vi "niDTS BT UTIL TV to Parameters.vi"(10 "BT Tx Parameters":T2={"Channel"=0, "Data Rate "=1, "Dut Tx Power"=0.0, "External Attenuation (dB)"=[0.0, 0.0, 0.0, 0.0], "Auto Level"=FALSE, "Packet type"=enum."DH1", "Payload Pattern"=enum."PN9", "Burst Sync"=enum."PREamble", "BD ADDRESS"=0, "Packet Length, bytes"=37, "ModAcc Measurement Paramaters"={"ModAcc Enable"=FALSE, "CFO Enable"=FALSE, "Character Select"=enum."DF1", "Averages"=1, "Averaging Mode"=enum."RMS", "Measurement Length"=-1, "Measurement Offset"=0}, "OBW Measurement Parameters"={"OBW Enable"=FALSE, "OBW Averages"=1, "Averaging Type"=enum."RMS", "Measurement Interval Mode"=enum."AUTO", "Measurement Interval Length (sec)"=0.005}, "TXP Measurement Parameters"={"TXP Power Enable"=FALSE, "TXP Averages"=1, "Averaging Type"=enum."RMS"}, "IBE  Measurement Parameters"={"IBE Enable"=FALSE, "IBE Averages"=1, "Averaging Type"=enum."RMS", "Numbe of Channels"=11, "Channel Mode"=enum."Centered", "Measurement Interval Mode"=enum."AUTO", "Measurement Interval Length (sec)"=0.005}, "Trace Enable"=FALSE, "Trigger"={"MinQuietTimeDuration (sec)"=0.0001, "TriggerDelay (sec)"=0.0, "TriggerEdge"=enum."RISing", "TriggerSource"=enum."RF0", "TriggerThreshold (dB)"=-20.0, "TriggerTimeout (sec)"=10.0}} {"BD ADDRESS" max=16777215 format="%.0x"}) -> (2 "niDTS BT DUT Parameters":T1={"Channel"=0, "Pattern"=enum."PN9", "Packet type"=enum."DH1", "Power"=0.0, "Report Period (ms)"=0.0, "BD Address"=0, "Data Rate"=enum."1", "Number of Packets"=1500, "Packet Length, bytes"=37} {"BD Address" format="%x"})   [LabVIEW 2015, in "niDTS BT.lvlib"]
uses:
  niDTS BT.lvlib
  Tests/Tx Test/Includes/niDTS BT Tx Test INC Parameters.ctl
  Includes/niDTS BT INC Packet Type.ctl
  Tests/Tx Test/Includes/niDTS BT Tx Test INC BD Payload Data.ctl
  Tests/Tx Test/Includes/niDTS BT Tx Test INC Modulation Characteristics.ctl
  Includes/niDTS BT INC OBW Measurement Parameters.ctl
  Includes/niDTS BT INC TXP Measurement Parameters.ctl
  Tests/EDR Tx Test/Includes/niDTS BT INC EDR IBE Measurement Parameters.ctl
  Includes/niDTS BT DUT INC Trigger.ctl
  Includes/niDTS BT DUT INC Parameters.ctl
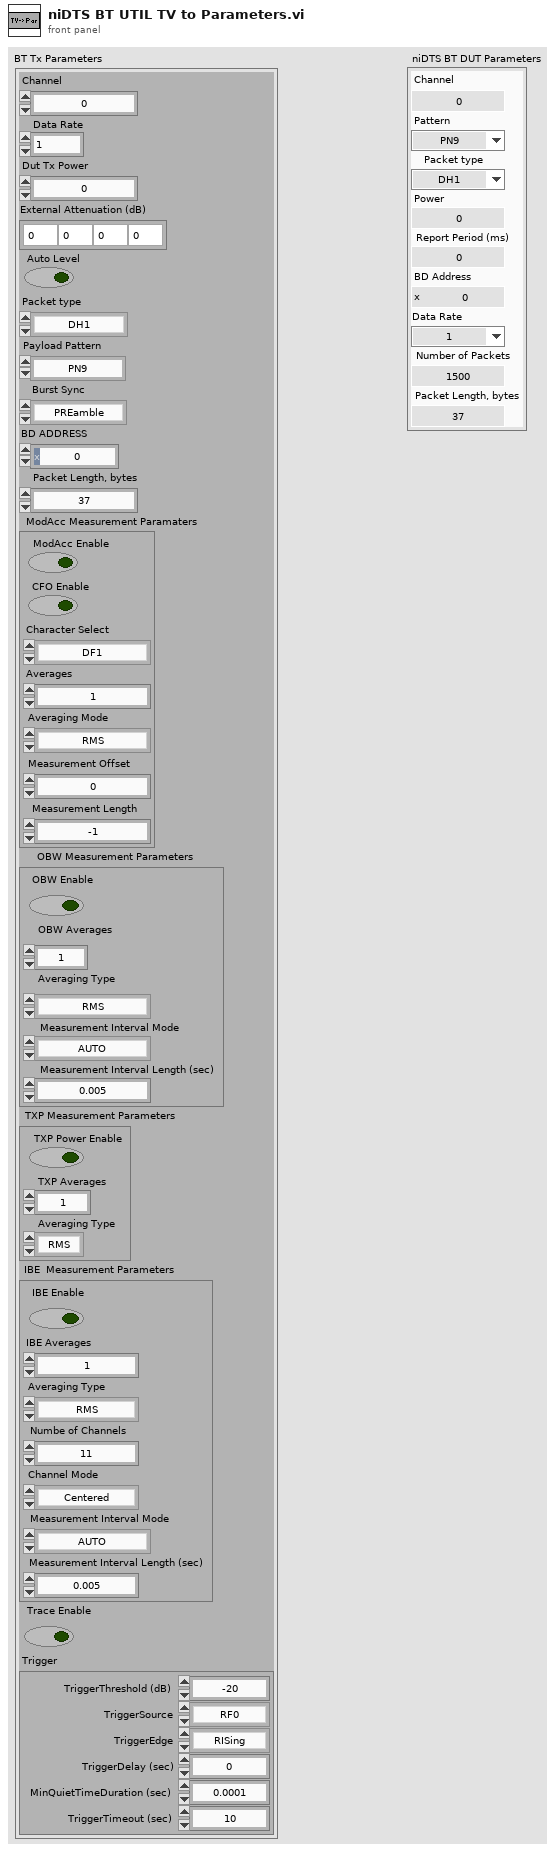
[diagram p1: front panel]
types:
  T1 = typedef "niDTS BT.lvlib/niDTS BT DUT INC Parameters.ctl" = cluster{"Channel":i32, "Pattern":enum16{"0", "1", "01", "00001111", "PN9"}, "Packet type":enum16{"NULL", "POLL", "FHS", "DM1", "DH1", "HV1", "HV2", "HV3", "EV3", "DV", "AUX1", "DM3", "DH3", "EV4", "EV5", "DM5", "DH5", "LE-TP"}, "Power":dbl, "Report Period (ms)":dbl, "BD Address":i64, "Data Rate":enum16{"1", "2", "3"}, "Number of Packets":i32, "Packet Length, bytes":i32}
  T2 = typedef "niDTS BT.lvlib/niDTS BT Tx Test INC Parameters.ctl" = cluster{"Channel":i32, "Data Rate ":i32, "Dut Tx Power":dbl, "External Attenuation (dB)":dbl[], "Auto Level":bool, "Packet type":T3, "Payload Pattern":T4, "Burst Sync":enum16{"NONE", "PREamble"}, "BD ADDRESS":u32, "Packet Length, bytes":i32, "ModAcc Measurement Paramaters":cluster{"ModAcc Enable":bool, "CFO Enable":bool, "Character Select":T5, "Averages":i32, "Averaging Mode":enum16{"RMS", "LOG", "SCALAR", "MAX", "MIN", "VECTOR"}, "Measurement Length":i32, "Measurement Offset":i32}, "OBW Measurement Parameters":T6, "TXP Measurement Parameters":T7, "IBE  Measurement Parameters":T8, "Trace Enable":bool, "Trigger":T9}
  T3 = typedef "niDTS BT.lvlib/niDTS BT INC Packet Type.ctl" = enum16{"NULL", "POLL", "FHS", "DM1", "DH1", "HV1", "HV2", "HV3", "EV3", "DV", "AUX1", "DM3", "DH3", "EV4", "EV5", "DM5", "DH5", "LE-TP"}
  T4 = typedef "niDTS BT.lvlib/niDTS BT Tx Test INC BD Payload Data.ctl" = enum16{"0", "1", "01", "00001111", "PN9", "AUTO"}
  T5 = typedef "niDTS BT.lvlib/niDTS BT Tx Test INC Modulation Characteristics.ctl" = enum16{"DF1", "DF2", "BOTH"}
  T6 = typedef "niDTS BT.lvlib/niDTS BT INC OBW Measurement Parameters.ctl" = cluster{"OBW Enable":bool, "OBW Averages":i32, "Averaging Type":enum16{"RMS", "LOG", "SCALAR", "MAX", "MIN", "VECTOR"}, "Measurement Interval Mode":enum16{"AUTO", "MANUAL"}, "Measurement Interval Length (sec)":dbl}
  T7 = typedef "niDTS BT.lvlib/niDTS BT INC TXP Measurement Parameters.ctl" = cluster{"TXP Power Enable":bool, "TXP Averages":i32, "Averaging Type":enum16{"RMS", "LOG", "SCALAR", "MAX", "MIN"}}
  T8 = typedef "niDTS BT.lvlib/niDTS BT INC EDR IBE Measurement Parameters.ctl" = cluster{"IBE Enable":bool, "IBE Averages":i32, "Averaging Type":enum16{"RMS", "LOG", "SCALAR", "MAX", "MIN", "VECTOR"}, "Numbe of Channels":i32, "Channel Mode":enum16{"InBand", "Centered"}, "Measurement Interval Mode":enum16{"AUTO", "MANUAL"}, "Measurement Interval Length (sec)":dbl}
  T9 = typedef "niDTS BT.lvlib/niDTS BT DUT INC Trigger.ctl" = cluster{"MinQuietTimeDuration (sec)":dbl, "TriggerDelay (sec)":dbl, "TriggerEdge":enum16{"RISing", "FALLing"}, "TriggerSource":enum16{"IMMediate", "RF0", "PFI0", "PFI1", "RTS0", "RTS1", "RTS2", "RTS3", "RTS4", "RTS5", "RTS6", "RTS7", "PXIStar", "SOFT"}, "TriggerThreshold (dB)":dbl, "TriggerTimeout (sec)":dbl}
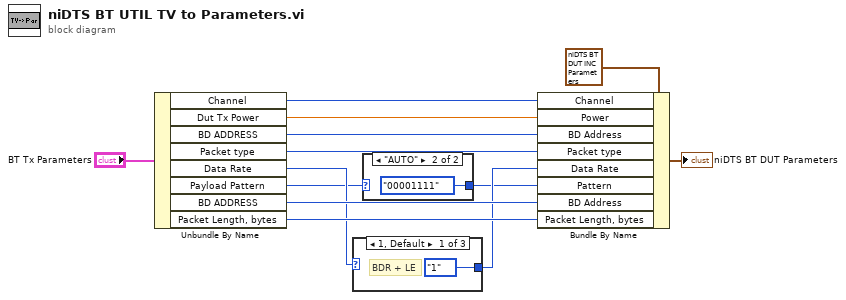
[diagram p0: block diagram]
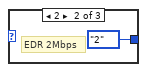
[diagram p3: hidden frame]
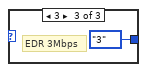
[diagram p4: hidden frame]
diagram:
  n1 = Unbundle By Name("BT Tx Parameters") -> ("Channel"=w10:i32, "Dut Tx Power"=w11:dbl, "BD ADDRESS"=w8:u32, "Packet type"=w6:T3, "Data Rate"=w4:i32, "Payload Pattern"=w2:T4, "BD ADDRESS"=w7:u32, "Packet Length, bytes"=w5:i32)
  n2 = case shown="1, Default" w4 {
    tunnel: [enum16{"1", "2", "3"}."1" ("Data Rate") enum16{"1", "2", "3"}."2" ("Data Rate") enum16{"1", "2", "3"}."3" ("Data Rate")] -> w3
    frame 1, Default {
      # "BDR + LE"
    }
    frame 2 {
      # "EDR 2Mbps"
    }
    frame 3 {
      # "EDR 3Mbps"
    }
  }
  n3 = case shown="\"AUTO\"" w2 {
    selector: w2 -> [w17 _]
    tunnel: [w17 enum16{"0", "1", "01", "00001111", "PN9"}."00001111" ("Pattern")] -> w1
    frame "0", Default {
    }
    frame "AUTO" {
    }
  }
  n4 = Bundle By Name(cluster=T1 {"Channel"=0, "Pattern"=enum."PN9", "Packet type"=enum."DH1", "Power"=0.0, "Report Period (ms)"=1000.0, "BD Address"=1500, "Data Rate"=enum."1", "Number of Packets"=1500, "Packet Length, bytes"=1500} ("niDTS BT DUT Parameters"), "Channel"=w10, "Power"=w11, "BD Address"=w8, "Packet type"=w6, "Data Rate"=w3, "Pattern"=w1, "BD Address"=w7, "Packet Length, bytes"=w5) -> (→"niDTS BT DUT Parameters":T1)
